vi "ParseSF.vi"(0 "data out":string) -> ()   [LabVIEW 2009]
panel:
  out "u2 7":sgl
  out "u1 5":sgl
  out "u2 6":sgl
  out "u2 5":sgl
  out "u1 4":sgl
  out "u2 4":sgl
  out "u1 3":sgl
  out "u2 3":sgl
  out "u1 2":sgl
  out "u2 2":sgl
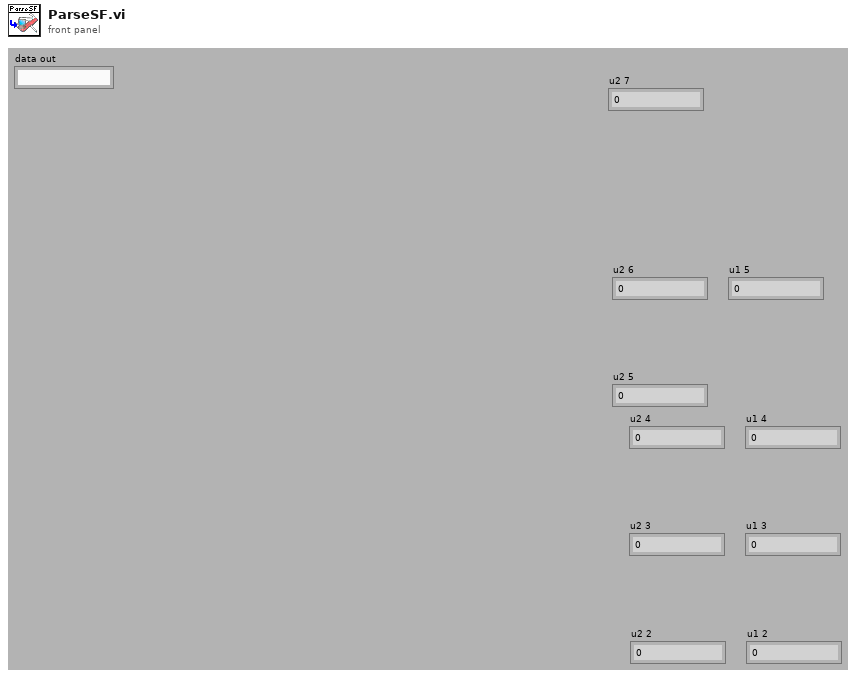
[diagram p1: front panel]
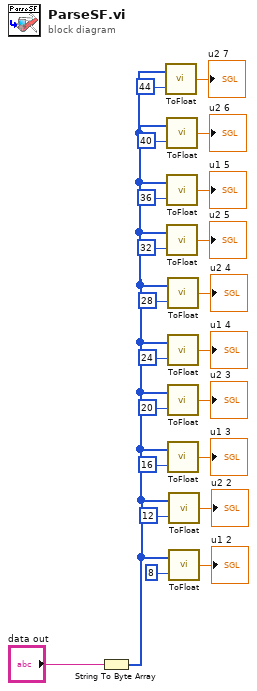
[diagram p0: block diagram]
diagram:
  n1 = String To Byte Array(string="data out") -> (unsigned byte array=w1:u8[])
  n2 = call "ToFloat.vi"("index"=44, "array"=w1) -> ("sp float"=→"u2 7":sgl)
  n3 = call "ToFloat.vi"("index"=40, "array"=w1) -> ("sp float"=→"u2 6":sgl)
  n4 = call "ToFloat.vi"("index"=36, "array"=w1) -> ("sp float"=→"u1 5":sgl)
  n5 = call "ToFloat.vi"("index"=32, "array"=w1) -> ("sp float"=→"u2 5":sgl)
  n6 = call "ToFloat.vi"("index"=28, "array"=w1) -> ("sp float"=→"u2 4":sgl)
  n7 = call "ToFloat.vi"("index"=24, "array"=w1) -> ("sp float"=→"u1 4":sgl)
  n8 = call "ToFloat.vi"("index"=20, "array"=w1) -> ("sp float"=→"u2 3":sgl)
  n9 = call "ToFloat.vi"("index"=16, "array"=w1) -> ("sp float"=→"u1 3":sgl)
  n10 = call "ToFloat.vi"("index"=12, "array"=w1) -> ("sp float"=→"u2 2":sgl)
  n11 = call "ToFloat.vi"("index"=8, "array"=w1) -> ("sp float"=→"u1 2":sgl)
